vi "_Run Engine.vi"() -> ()   [LabVIEW 2012]
uses:
  Type/_Run State.ctl
  Type/_Data Operation.ctl
  Type/_File Command.ctl
  Type/_RT Command.ctl
  Configuration/_Global Configuration.vi
  Server/_Server Global.vi
panel:
  out "size(s)":i32
  out "first subarray":i32[](array[numeric])
  out "error":string
  out "Occurance timed out":bool
  out "Done":bool
  out "error out":errorcluster
  out "Remaining Scans":i32
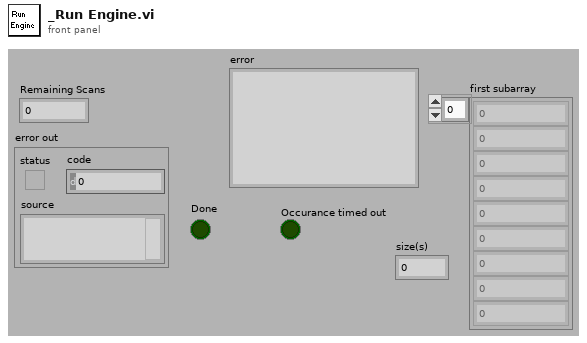
[diagram p1: front panel]
types:
  T1 = typedef "_Run State.ctl" = enum16{"Init", "Update", "Start", "End", "Error"}
  T2 = typedef "_Data Operation.ctl" = enum8{"Initialize", "Get Data", "Set Data", "Close"}
  T3 = typedef "_File Command.ctl" = enum16{"No Command", "Open", "Open Read", "Write", "Get Spectrum", "Close"}
  T4 = typedef "_RT Command.ctl" = enum16{"Start", "Stop", "Runtime Update", "Get Data", "Get Info", "Get Status", "Get Param", "Get Config", "Get Table", "Read ADC", "Set Oscillator", "Update Config", "Update Table", "Set All Pol", "Set Pol and DC", "Set Max Mass", "Toggle RP", "Toggle EL", "Set PIC", "Initialize Turbo", "Send Turbo Comm", "Close Turbo", "P1", "P2", "P3", "Send Serial", "Set LC Out", "Get LC In", "Read VAC", "Test Table", "Toggle Power", "Get Startup", "Set Startup", "Get ADC Table", "Set ADC Table", "Get Brief Status", "Get Detail Status", "Auxiliary Update", "Set CC Logics", "Set CC Input Logics", "Ignore Error"}
  T5 = typedef "_XML Expt.ctl" = cluster{"StartT(mS)":i32, "#Cycles":i32, "PauseT(uS)":i32, "ScanType":i32, "Polarity":u8, "FixedMass":dbl, "DelayT(mS)":i32, "Active Ch":T6[], "Mass Range":T7[]}
  T6 = typedef "_XML Lens.ctl" = cluster{"Value":dbl, "ChID":u8}
  T7 = typedef "_Mass Range Property.ctl" = cluster{"Start":dbl, "Stop":dbl, "Step Size":dbl, "Steps":i32, "Dwell":dbl, "Parameters":T8[], "Res":T9}
  T8 = typedef "_Mass Range Parameters.ctl" = cluster{"Name":string, "Ch#":u8, "StartV":dbl, "StopV":dbl, "StepV":dbl, "Index":u8}
  T9 = typedef "_RT Res Type.ctl" = u16
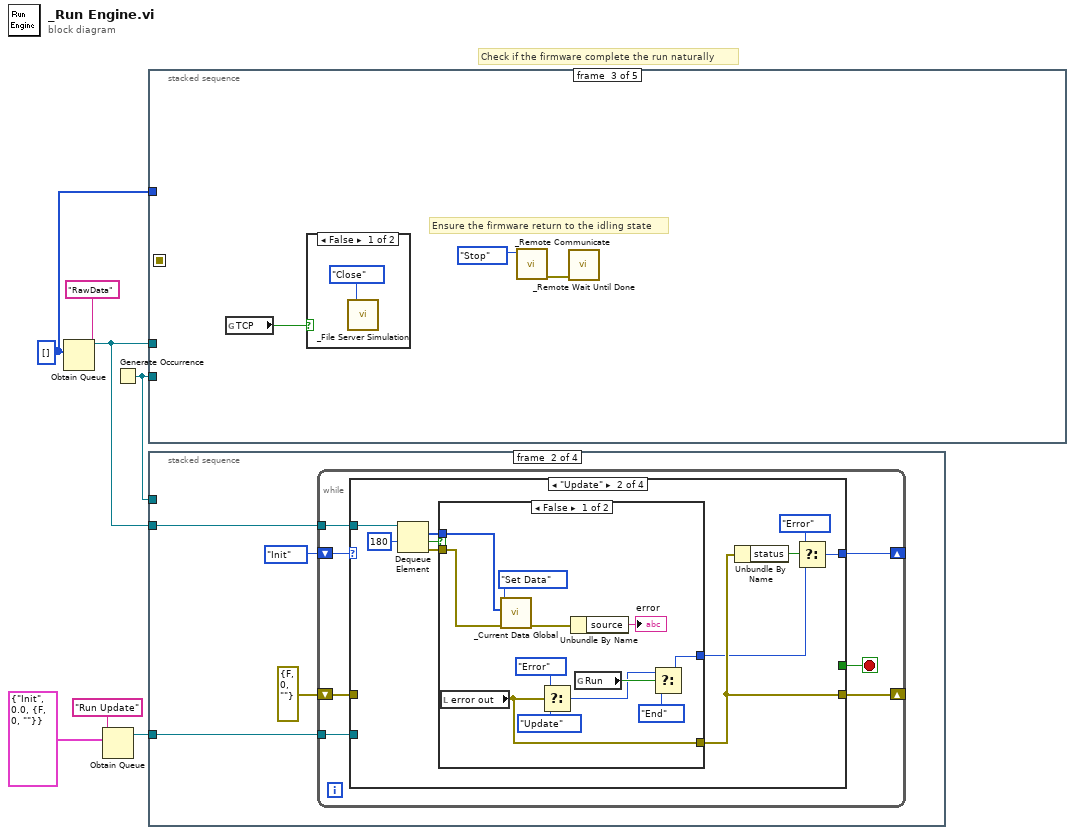
[diagram p0: block diagram]
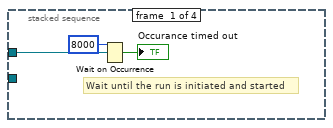
[diagram p2: hidden frame]
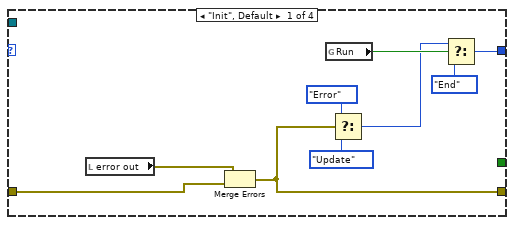
[diagram p3: hidden frame]
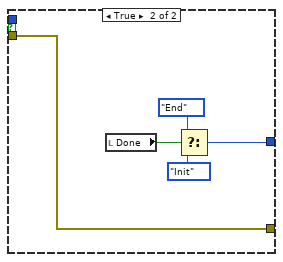
[diagram p4: hidden frame]
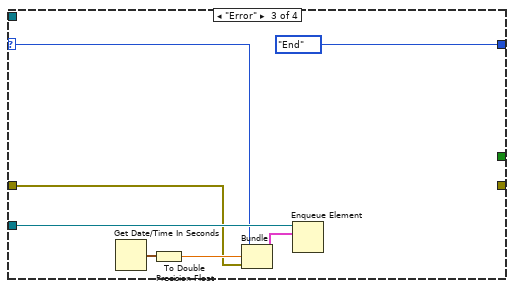
[diagram p5: hidden frame]
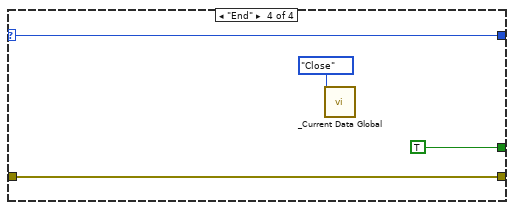
[diagram p6: hidden frame]
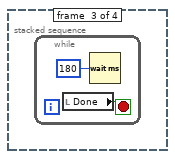
[diagram p7: hidden frame]
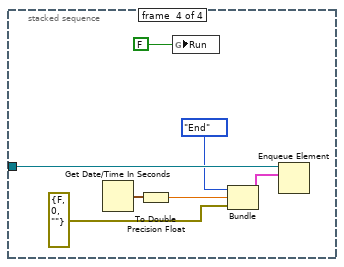
[diagram p8: hidden frame]
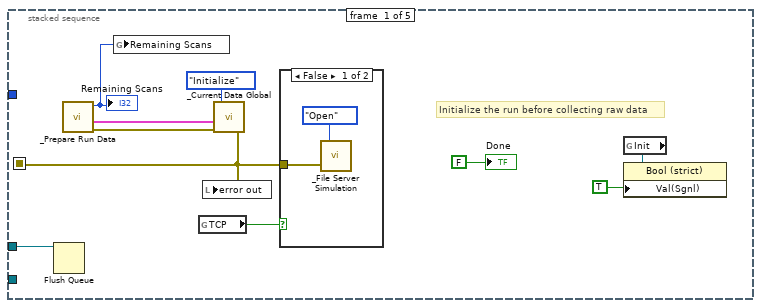
[diagram p9: hidden frame]
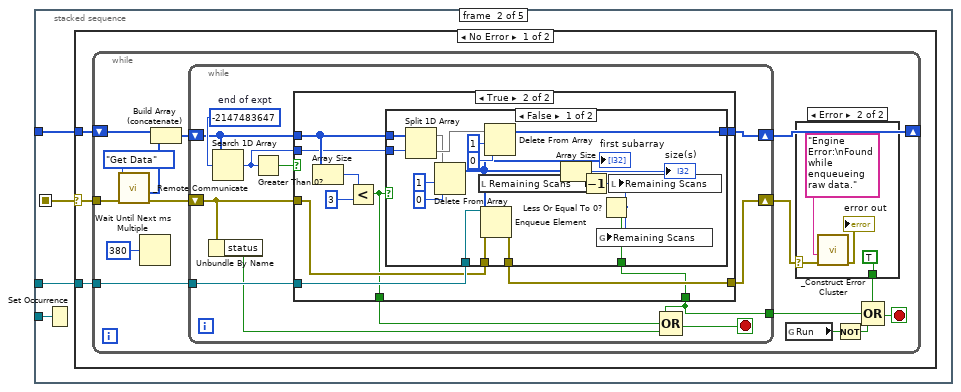
[diagram p11: hidden frame]
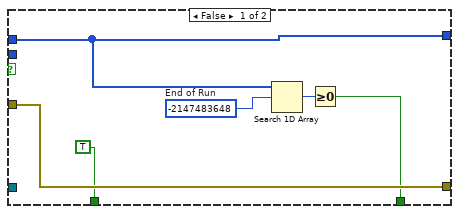
[diagram p12: hidden frame]
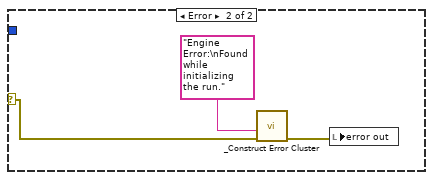
[diagram p15: hidden frame]
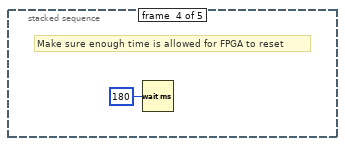
[diagram p17: hidden frame]
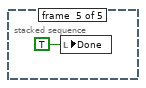
[diagram p18: hidden frame]
diagram:
  w4 = i32[] []
  # "Check if the firmware complete the run naturally"
  n1 = Obtain Queue(name (unnamed)="RawData", element data type=w4) -> (queue out=w5:refnum<queue>)  [unwired: 3 in, 2 out]
  n2 = Obtain Queue(name (unnamed)="Run Update", element data type=cluster{T1, dbl, "error out":errorcluster} {enum."Init", 0.0, "error out"={"status"=FALSE, "code"=0, "source"=""}}) -> (queue out=w2:refnum<queue>)  [unwired: 3 in, 2 out]
  n3 = Generate Occurrence() -> (w6:refnum<k4>)
  n4 = stacked-sequence {
    seq-local: [w8 _ _ _ _] -> [_ w21 _ _ _]
    tunnel: w6 -> [_ w22 _ _ _]
    tunnel: w5 -> [w17 w23 _ _ _]
    tunnel: w4 -> [_ w20 _ _ _]
    frame #0 {
      # "Initialize the run before collecting raw data"
      n5 = Flush Queue(queue=w17) -> ()  [unwired: 1 in, 3 out]
      n6 = call "_Prepare Run Data.vi"() -> ("error out"=w12:errorcluster, "AcqMethod"=w11:T5[], "Scans"=w10:i32)  [unwired: 1 in, 8 out]
      "Remaining Scans" <- w10
      n7 = global write "_Server Global.vi" "Remaining Scans"(w10) -> ()
      n8 = global read "_Global Configuration.vi" "TCP"() -> (w9:bool)
      n9 = call "_Current Data Global.vi"("error in (no error)"=w12, "AcqMethod"=w11, "Operation"=_Data_Operation."Initialize") -> ("error out"=w8:errorcluster)  [unwired: 1 in, 3 out]
      n10 = local write "error out"(w8) -> ()
      n11 = case shown="False" w9 {
        tunnel: w8 -> [w18 _]
        frame False {
          n12 = call "_File Server Simulation.vi"("ErrorIn"=w18, "FileCommand"=_File_Command."Open") -> ()  [unwired: 2 out]
        }
        frame True {
        }
      }
      n13 = global read "_Global Configuration.vi" "Init"() -> (w15:refnum<vi>)
      n14 = property class="Bool (strict)"(reference=w15, "Val(Sgnl)"=TRUE ("Value (Signaling)")) -> ()  [unwired: 1 in, 2 out]
      "Done" <- FALSE ("Done")
    }
    frame #1 {
      n15 = Set Occurrence(w22) -> ()
      n16 = case shown="No Error" w21 {
        selector: w21 -> [w25 w93]
        tunnel: w23 -> [w26 _]
        tunnel: w20 -> [w24 _]
        frame No Error {
          n17 = while {
            tunnel: w26 -> [w40]
            tunnel: w25 -> [w36]
            shift-right: [w33] -> _
            shift-left: w24 -> [w31]
            stop <- w39 stop-if-true
            n18 = call "_Remote Communicate.vi"("error in (no error)"=w36, "Command"=_RT_Command."Get Data") -> ("error out"=w29:errorcluster, "Data Array"=w28:i32[])  [unwired: 4 in, 2 out]
            n19 = Wait Until Next ms Multiple(millisecond multiple=u32 380) -> ()  [unwired: 1 out]
            n20 = Build Array (concatenate)(w31, w28) -> (w30:i32[])
            n21 = while {
              tunnel: w40 -> [w53]
              tunnel: [w45] -> w32
              shift-right: [w51] -> w33
              shift-left: w30 -> [w49]
              shift-right: [w52] -> w35
              shift-left: w29 -> [w47]
              stop <- w43 stop-if-true
              w50 = -2147483647  # end of expt
              n22 = Unbundle By Name(w47) -> ("status"=w44:bool)
              n23 = Search 1D Array(1D array=w49, element=w50) -> (index of element=w48:i32)  [unwired: 1 out]
              n24 = Greater Than 0?(x=w48) -> (x > 0?=w46:bool)
              n25 = case shown="True" w46 {
                tunnel: w47 -> [w59 w67]
                tunnel: w53 -> [_ w68]
                tunnel: [w59 w66] -> w52
                tunnel: w49 -> [w56 w62]
                tunnel: [w56 w69] -> w51
                tunnel: [w55 w65] -> w45
                tunnel: w48 -> [_ w61]
                tunnel: [TRUE w60] -> w42
                frame False {
                  w57 = -2147483648  # End of Run
                  n26 = Search 1D Array(1D array=w56, element=w57) -> (index of element=w58:i32)  [unwired: 1 out]
                  n27 = Greater Or Equal To 0?(x=w58) -> (x >= 0?=w55:bool)
                }
                frame True {
                  n28 = Array Size(array=w62) -> (size(s)=w64:i32)
                  n29 = Less?(x=w64, y=3) -> (x < y?=w60:bool)
                  n30 = case shown="False" w60 {
                    tunnel: w62 -> [w86 w87]
                    tunnel: w61 -> [w85 _]
                    tunnel: [w78 w87] -> w69
                    tunnel: w68 -> [w81 _]
                    tunnel: w67 -> [w80 w88]
                    tunnel: [w79 w88] -> w66
                    tunnel: [w71 _] -> w65
                    frame False {
                      n31 = Split 1D Array(array=w86, index=w85) -> (first subarray=w73:i32[], second subarray=w83:i32[])
                      n32 = Delete From Array(array=w73, length=1, index=0) -> (array with subset deleted=w72:i32[])  [unwired: 1 out]
                      "first subarray" <- w72
                      n33 = local read "Remaining Scans"() -> (w77:i32)
                      n34 = Enqueue Element(queue=w81, element=w72, error in (no error)=w80) -> (error out=w79:errorcluster)  [unwired: 3 out]
                      n35 = Delete From Array(array=w83, length=1, index=0) -> (array with subset deleted=w78:i32[])  [unwired: 1 out]
                      n36 = Array Size(array=w72) -> (size(s)=→"size(s)":i32)
                      n37 = Decrement(x=w77) -> (x-1=w70:i32)
                      n38 = global write "_Server Global.vi" "Remaining Scans"(w70) -> ()
                      n39 = Less Or Equal To 0?(x=w70) -> (x <= 0?=w71:bool)
                      n40 = local write "Remaining Scans"(w70) -> ()
                    }
                    frame True {
                    }
                  }
                }
              }
              n41 = Compound Arithmetic op=OR(w45, w42, w44) -> (w43:bool)
            }
            n42 = global read "_Global Configuration.vi" "Run"() -> (w38:bool)
            n43 = case shown="Error" w35 {
              selector: w35 -> [_ w92]
              tunnel: [_ TRUE] -> w34
              frame No Error {
              }
              frame Error {
                n44 = call "_Construct Error Cluster.vi"("error in"=w92, "reason"="Engine Error:\nFound while enqueueing raw data." ("format string")) -> ("error out"=→"error out":errorcluster)  [unwired: 2 in, 3 out]
              }
            }
            n45 = Not(x=w38) -> (.not. x?=w37:bool)
            n46 = Compound Arithmetic op=OR(w34, w32, w37) -> (w39:bool)
          }
        }
        frame Error {
          n47 = call "_Construct Error Cluster.vi"("error in"=w93, "reason"="Engine Error:\nFound while initializing the run." ("format string")) -> ("error out"=w94:errorcluster)  [unwired: 2 in, 3 out]
          n48 = local write "error out"(w94) -> ()
        }
      }
    }
    frame #2 {
      # "Ensure the firmware return to the idling state"
      n49 = global read "_Global Configuration.vi" "TCP"() -> (w96:bool)
      n50 = case shown="False" w96 {
        frame False {
          n51 = call "_File Server Simulation.vi"("FileCommand"=_File_Command."Close") -> ()  [unwired: 1 in, 2 out]
        }
        frame True {
        }
      }
      n52 = call "_Remote Communicate.vi"("Command"=_RT_Command."Stop") -> ("error out"=w98:errorcluster)  [unwired: 5 in, 3 out]
      n53 = call "_Remote Wait Until Done.vi"("error IO"=w98) -> ()  [unwired: 1 in, 2 out]
    }
    frame #3 {
      # "Make sure enough time is allowed for FPGA to reset"
      n54 = Wait (ms)(milliseconds to wait=u32 180) -> ()  [unwired: 1 out]
    }
    frame #4 {
      n55 = local write "Done"(TRUE ("Done")) -> ()
    }
  }
  n56 = stacked-sequence {
    tunnel: w6 -> [w104 _ _ _]
    tunnel: w5 -> [_ w107 _ _]
    tunnel: w2 -> [_ w106 _ w168]
    frame #0 {
      # "Wait until the run is initiated and started"
      n57 = Wait on Occurrence(2:w104, 3:8000 ("ms timeout (-1)")) -> (0:→"Occurance timed out":bool)  [unwired: 1 out]
    }
    frame #1 {
      n58 = while {
        shift-right: [w114] -> _
        shift-left: _Run_State."Init" -> [w115]
        shift-right: [w113] -> _
        shift-left: errorcluster {"status"=FALSE, "code"=0, "source"=""} ("error out") -> [w112]
        tunnel: w106 -> [w110]
        tunnel: w107 -> [w109]
        stop <- w111 stop-if-true
        n59 = case shown="\"Update\"" w115 {
          selector: w115 -> [_ _ w153 w161]
          tunnel: [w118 w132 _Run_State."End" w161] -> w114
          tunnel: [w121 w126 _ w160] -> w113
          tunnel: w112 -> [w123 _ w152 w160]
          tunnel: [_ _ _ TRUE] -> w111
          tunnel: w110 -> [_ _ w154 _]
          tunnel: w109 -> [_ w131 _ _]
          frame "Init", Default {
            n60 = local read "error out"() -> (w122:errorcluster)
            n61 = Merge Errors(w122, w123) -> (w121:errorcluster)
            n62 = global read "_Global Configuration.vi" "Run"() -> (w117:bool)
            n63 = Select(t=_Run_State."Error", s=w121, f=_Run_State."Update") -> (s? t:f=w116:T1)
            n64 = Select(t=w116, s=w117, f=_Run_State."End") -> (s? t:f=w118:T1)
          }
          frame "Update" {
            n65 = Dequeue Element(queue=w131, timeout in ms (-1)=180) -> (element=w127:i32[], timed out?=w129:bool, error out=w128:errorcluster)  [unwired: 1 in, 1 out]
            n66 = case shown="False" w129 {
              tunnel: w128 -> [w138 w151]
              tunnel: w127 -> [w137 _]
              tunnel: [w139 w151] -> w126
              tunnel: [w140 w147] -> w125
              frame False {
                n67 = local read "error out"() -> (w139:errorcluster)
                n68 = call "_Current Data Global.vi"("error in (no error)"=w138, "Spectrum in"=w137, "Operation"=_Data_Operation."Set Data") -> ("error out"=w135:errorcluster)  [unwired: 1 in, 3 out]
                n69 = Select(t=_Run_State."Error", s=w139, f=_Run_State."Update") -> (s? t:f=w141:T1)
                n70 = Unbundle By Name(w135) -> ("source"=→"error":string)
                n71 = global read "_Global Configuration.vi" "Run"() -> (w142:bool)
                n72 = Select(t=w141, s=w142, f=_Run_State."End") -> (s? t:f=w140:T1)
              }
              frame True {
                n73 = local read "Done"() -> (w150:bool)
                n74 = Select(t=_Run_State."End", s=w150, f=_Run_State."Init") -> (s? t:f=w147:T1)
              }
            }
            n75 = Unbundle By Name(w126) -> ("status"=w133:bool)
            n76 = Select(t=_Run_State."Error", s=w133, f=w125) -> (s? t:f=w132:T1)
          }
          frame "Error" {
            n77 = Get Date/Time In Seconds() -> (seconds since 1Jan1904=w157:timestamp)
            n78 = To Double Precision Float(number=w157) -> (double precision float=w155:dbl)
            n79 = Bundle(w153, w155, "error out"=w152) -> (w156:cluster{T1, dbl, "error out":errorcluster})  [unwired: 1 out]
            n80 = Enqueue Element(queue=w154, element=w156) -> ()  [unwired: 1 in, 4 out]
          }
          frame "End" {
            n81 = call "_Current Data Global.vi"("Operation"=_Data_Operation."Close") -> ()  [unwired: 3 in, 4 out]
          }
        }
      }
    }
    frame #2 {
      n82 = while {
        stop <- w164 stop-if-true
        n83 = local read "Done"() -> (w164:bool)
        n84 = Wait (ms)(milliseconds to wait=u32 180) -> ()  [unwired: 1 out]
      }
    }
    frame #3 {
      n85 = Get Date/Time In Seconds() -> (seconds since 1Jan1904=w171:timestamp)
      n86 = To Double Precision Float(number=w171) -> (double precision float=w169:dbl)
      n87 = global write "_Global Configuration.vi" "Run"(FALSE ("Update")) -> ()
      n88 = Bundle(_Run_State."End", w169, "error out"=errorcluster {"status"=FALSE, "code"=0, "source"=""}) -> (w170:cluster{T1, dbl, "error out":errorcluster})  [unwired: 1 out]
      n89 = Enqueue Element(queue=w168, element=w170) -> ()  [unwired: 1 in, 4 out]
    }
  }
